vi "mWADC_init.vi"(8 "err_in":errorcluster, 11 "mWADC_Port":refnum<visa-resource-name>) -> (0 "error out":errorcluster, 3 "reference out":refnum<visa-resource-name>)   [LabVIEW 2019]
uses:
  <vilib>/Instr/_visa.llb/VISA Flush IO Buffer Mask.ctl
panel:
  in  "Mask":T1=16 items=["Flush Receive Buffer"=16, "Write Transmit Buffer to Device"=32, "Flush Receive Buffer (No I/O)"=64, "Flush Transmit Buffer"=128]
  in  "Message Based Settings:Suppress End Enable":bool
  in  "Message Based Settings:Send End Enable":bool=TRUE
  in  "Message Based Settings:Termination Character Enable":bool=TRUE
  in  "Serial Settings:End Mode for Writes":u16(ring)=2 items=["None", "Last Bit", "TermChar", "Break"]
  in  "Serial Settings:End Mode for Reads":u16(ring)=2 items=["None", "Last Bit", "TermChar"]
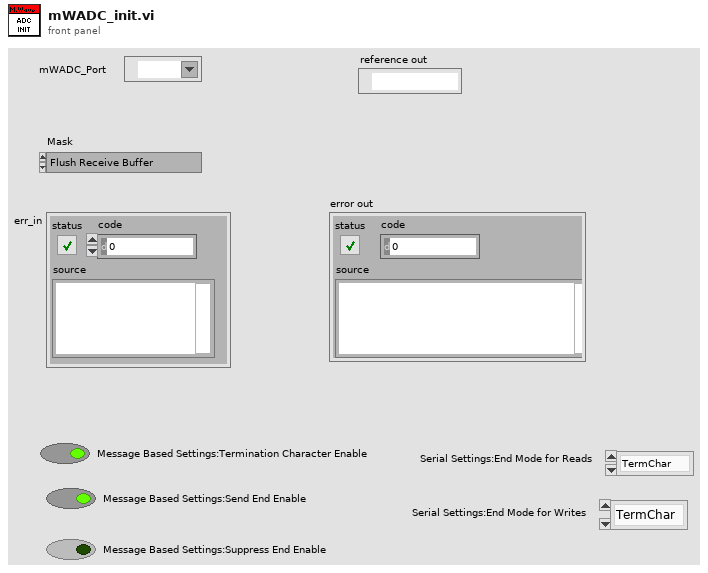
[diagram p1: front panel]
types:
  T1 = typedef "VISA Flush IO Buffer Mask.ctl" = u16
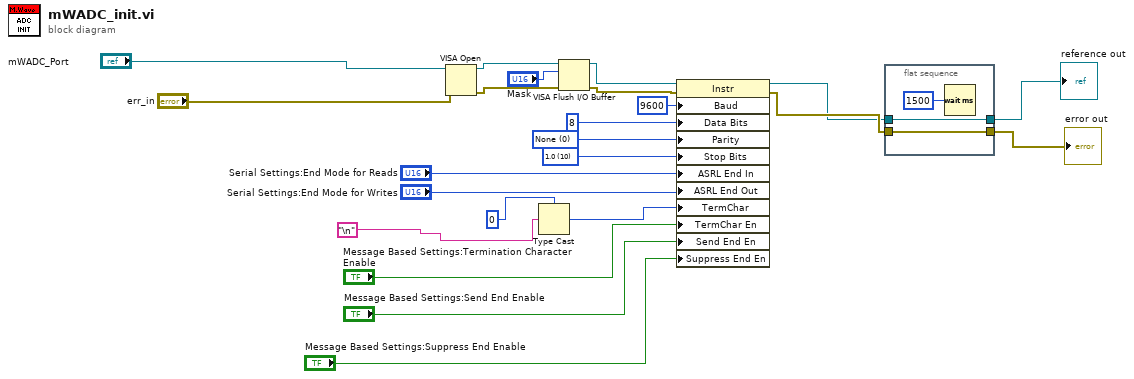
[diagram p0: block diagram]
diagram:
  w20 = u16 10 items=["1.0"=10, "1.5"=15, "2.0"=20] ("Serial Settings:Stop Bits")
  w21 = u16 0 items=["None", "Odd", "Even", "Mark", "Space"] ("Serial Settings:Parity")
  n1 = VISA Open(error in (no error)="err_in", VISA resource name="mWADC_Port") -> (VISA resource name=w10:refnum<visa-resource-name>, error out=w7:errorcluster)  [unwired: 3 in]
  n2 = Type Cast(type=u8 0, x="\n") -> (*(type *) &x=w16:u8)
  n3 = VISA Flush I/O Buffer(VISA resource name=w10, mask (16)="Mask", error in (no error)=w7) -> (VISA resource name out=w9:refnum<visa-resource-name>, error out=w8:errorcluster)
  n4 = property class="Instr"(reference=w9, error in=w8, "Baud"=u32 9600 ("Serial Settings:Baud Rate"), "Data Bits"=u16 8 ("Serial Settings:Data Bits"), "Parity"=w21, "Stop Bits"=w20, "ASRL End In"="Serial Settings:End Mode for Reads", "ASRL End Out"="Serial Settings:End Mode for Writes", "TermChar"=w16, "TermChar En"="Message Based Settings:Termination Character Enable", "Send End En"="Message Based Settings:Send End Enable", "Suppress End En"="Message Based Settings:Suppress End Enable") -> (reference out=w1:refnum<visa-resource-name>, error out=w4:errorcluster)
  n5 = flat-sequence {
    tunnel: [w25] -> w2
    tunnel: w1 -> [w25]
    tunnel: w4 -> [w24]
    tunnel: [w24] -> w3
    frame #0 {
      n6 = Wait (ms)(milliseconds to wait=u32 1500) -> ()  [unwired: 1 out]
    }
  }
  "error out" <- w3
  "reference out" <- w2
